vi "Send REGISTER.vi"(8 "REGISTER request data":T1, 9 "Message Loop Shift Register Data":T2, 10 "error in (no error)":errorcluster, 11 "WAMP Client in":refnum<class "WAMP Client.lvclass">) -> (1 "Message Loop Shift Register Data":T2, 2 "error out":errorcluster, 3 "WAMP Client out":refnum<class "WAMP Client.lvclass">)   [LabVIEW 2020, in "WAMP Client.lvclass"]
uses:
  <userlib>/lvwamp/WAMP Client/WAMP Client.lvclass
  <userlib>/lvwamp/WAMP Message Codes.ctl
  <userlib>/lvwamp/WAMP Client/WAMP Client.lvclass/WAMP Client.ctl
  <vilib>/numeric/sub_Random U32.vi
  <userlib>/lvwamp/WAMP Client/TypeDef/WAMP Error Payload.ctl
  <userlib>/lvwamp/WAMP Client/TypeDef/REGISTERED or ERROR payload.ctl
  <userlib>/lvwamp/WAMP Client/TypeDef/INVOCATION payload.ctl
  <userlib>/lvwamp/WAMP Client/TypeDef/REGISTER Request Data.ctl
  <userlib>/lvwamp/WAMP Client/TypeDef/Message Loop Shift Reg Data.ctl
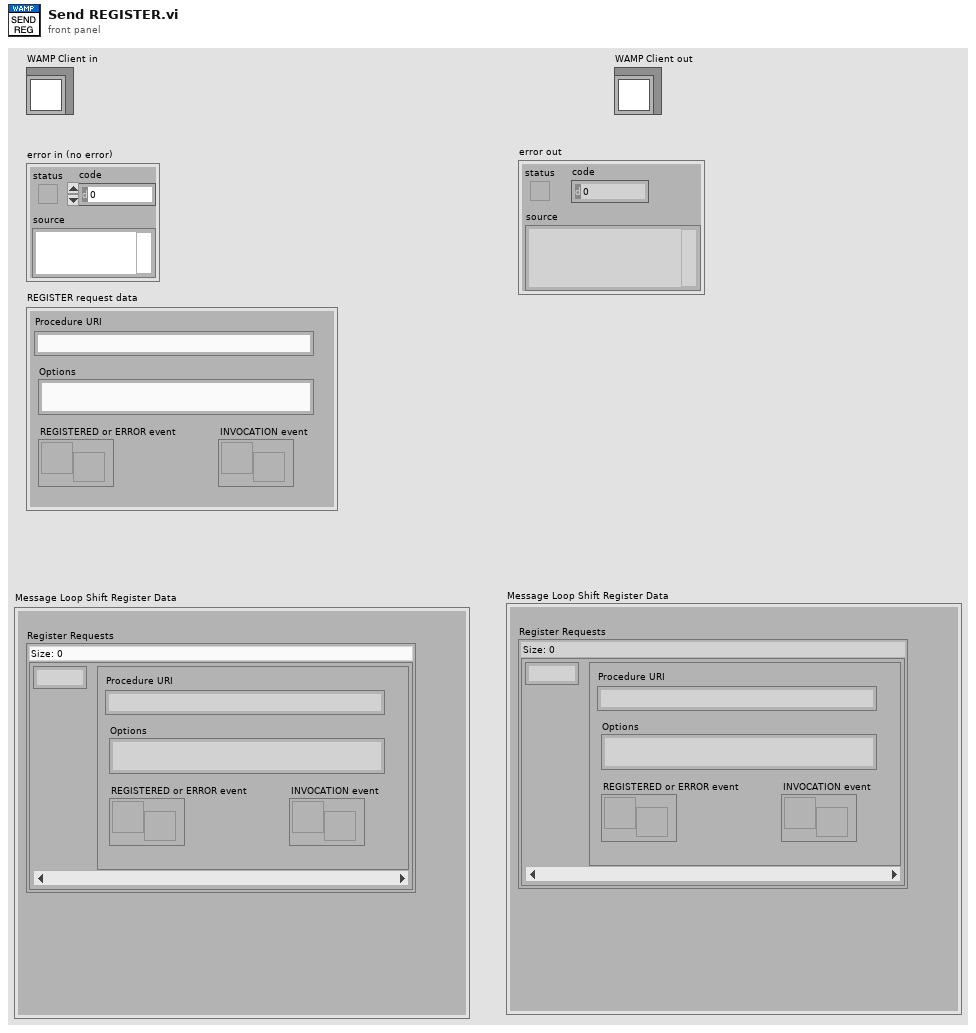
[diagram p1: front panel]
types:
  T1 = typedef "WAMP Client.lvclass/REGISTER Request Data.ctl" = cluster{"Procedure URI":string, "Options":string, "REGISTERED or ERROR event":refnum<user-event>, "INVOCATION event":refnum<user-event>}
  T2 = typedef "WAMP Client.lvclass/Message Loop Shift Reg Data.ctl" = cluster{"Register Requests":map{u32, T1}}
  T3 = typedef "WAMP Client.lvclass/WAMP Message Codes.ctl" = u16
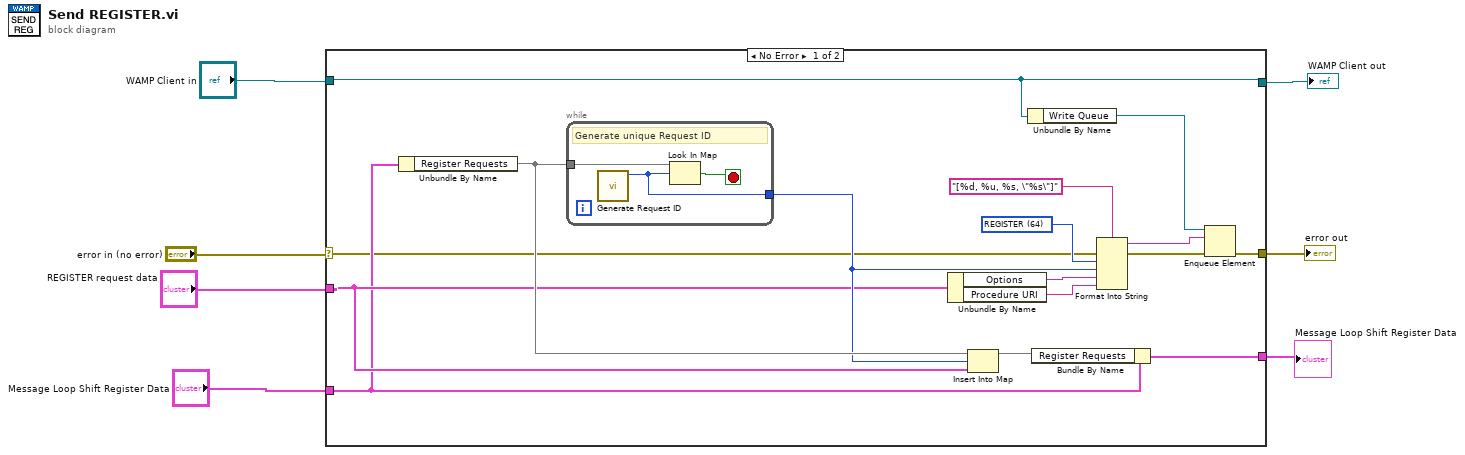
[diagram p0: block diagram]
diagram:
  n1 = case shown="No Error" "error in (no error)" {
    selector: "error in (no error)" -> [w8 w29]
    tunnel: [w18 w29] -> w6
    tunnel: [w19 w28] -> w4
    tunnel: "WAMP Client in" -> [w19 w28]
    tunnel: "REGISTER request data" -> [w12 _]
    tunnel: "Message Loop Shift Register Data" -> [w11 w27]
    tunnel: [w9 w27] -> w1
    frame No Error {
      w20 = T3 64 items=["HELLO"=1, "WELCOME"=2, "ABORT"=3, "GOODBYE"=6, "ERROR"=8, "PUBLISH"=16, "PUBLISHED"=17, "SUBSCRIBE"=32, "SUBSCRIBED"=33, "UNSUBSCRIBE"=34, "UNSUBSCRIBED"=35, "EVENT"=36, "CALL"=48, "RESULT"=59, "REGISTER"=64, "REGISTERED"=65, "UNREGISTER"=66, "UNREGISTERED"=67, "INVOCATION"=68, "YIELD"=70] ("Message Codes")
      n2 = Unbundle By Name(w11) -> ("Register Requests"=w14:map{u32, T1})
      n3 = while {
        tunnel: w14 -> [w26]
        tunnel: [w24] -> w13
        stop <- w25 stop-if-true
        # "Generate unique Request ID"
        n4 = call <userlib>:"Generate Request ID.vi"() -> ("Generate Request ID"=w24:u32)  [unwired: 11 in]
        n5 = Look In Map(map=w26, key=w24) -> (key not found?=w25:bool)  [unwired: 1 in, 1 out]
      }
      n6 = Unbundle By Name(w12) -> ("Options"=w16:string, "Procedure URI"=w15:string)
      n7 = Insert Into Map(map in=w14, key=w13, value=w12) -> (map out=w10:map{u32, T1})  [unwired: 2 out]
      n8 = Unbundle By Name(w19) -> ("Write Queue"=w17:refnum<queue>)
      n9 = Bundle By Name(cluster=w11, "Register Requests"=w10) -> (w9:T2)
      n10 = Format Into String(format string="[%d, %u, %s, \"%s\"]" ("element"), error in=w8, w20, w13, w16, w15) -> (resulting string=w22:string, error out=w23:errorcluster)  [unwired: 1 in]
      n11 = Enqueue Element(queue=w17, element=w22, error in (no error)=w23) -> (error out=w18:errorcluster)  [unwired: 1 in, 2 out]
    }
    frame Error {
    }
  }
  "error out" <- w6
  "WAMP Client out" <- w4
  "Message Loop Shift Register Data" <- w1
